vi "MainDisplay.vi"   [LabVIEW 2013]
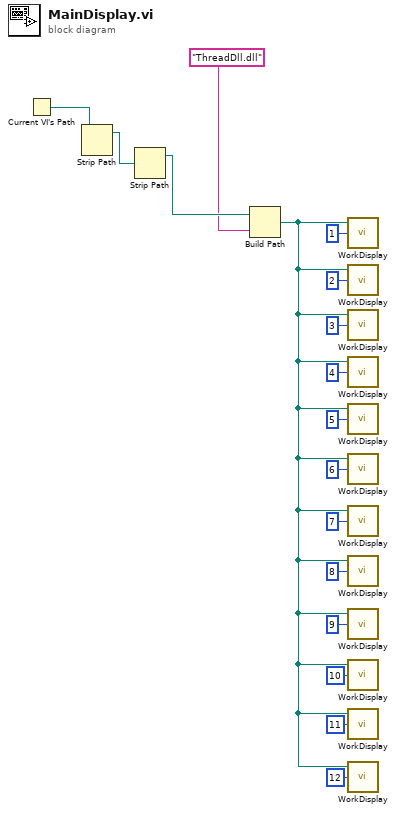
[diagram p0: block diagram]
diagram:
  n1 = Current VI's Path() -> (path=w17:path)
  n2 = Strip Path(path=w17) -> (stripped path=w1:path)  [unwired: 1 out]
  n3 = Strip Path(path=w1) -> (stripped path=w16:path)  [unwired: 1 out]
  n4 = Build Path(base path=w16, name or relative path="ThreadDll.dll") -> (appended path=w13:path)
  n5 = call "WorkDisplay.vi"("idNumber"=i64 1, "Dll Path"=w13) -> ()  [unwired: 3 in, 1 out]
  n6 = call "WorkDisplay.vi"("idNumber"=i64 2, "Dll Path"=w13) -> ()  [unwired: 3 in, 1 out]
  n7 = call "WorkDisplay.vi"("idNumber"=i64 3, "Dll Path"=w13) -> ()  [unwired: 3 in, 1 out]
  n8 = call "WorkDisplay.vi"("idNumber"=i64 4, "Dll Path"=w13) -> ()  [unwired: 3 in, 1 out]
  n9 = call "WorkDisplay.vi"("idNumber"=i64 5, "Dll Path"=w13) -> ()  [unwired: 3 in, 1 out]
  n10 = call "WorkDisplay.vi"("idNumber"=i64 6, "Dll Path"=w13) -> ()  [unwired: 3 in, 1 out]
  n11 = call "WorkDisplay.vi"("idNumber"=i64 7, "Dll Path"=w13) -> ()  [unwired: 3 in, 1 out]
  n12 = call "WorkDisplay.vi"("idNumber"=i64 8, "Dll Path"=w13) -> ()  [unwired: 3 in, 1 out]
  n13 = call "WorkDisplay.vi"("idNumber"=i64 9, "Dll Path"=w13) -> ()  [unwired: 3 in, 1 out]
  n14 = call "WorkDisplay.vi"("idNumber"=i64 10, "Dll Path"=w13) -> ()  [unwired: 3 in, 1 out]
  n15 = call "WorkDisplay.vi"("idNumber"=i64 11, "Dll Path"=w13) -> ()  [unwired: 3 in, 1 out]
  n16 = call "WorkDisplay.vi"("idNumber"=i64 12, "Dll Path"=w13) -> ()  [unwired: 3 in, 1 out]
